vi "invert cluster.vi"(11 "subcarrier channels":T1) -> (2 "subcarrier channels out":T1)   [LabVIEW 2020]
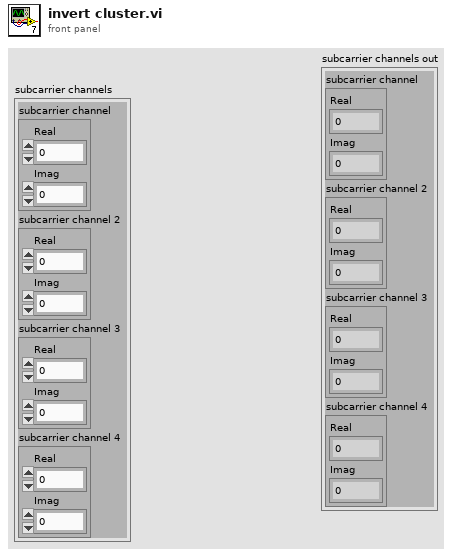
[diagram p1: front panel]
types:
  T1 = cluster{"subcarrier channel":cluster{"Real":fxp<+/-,25,4>, "Imag":fxp<+/-,25,4>}, "subcarrier channel 2":cluster{"Real":fxp<+/-,25,4>, "Imag":fxp<+/-,25,4>}, "subcarrier channel 3":cluster{"Real":fxp<+/-,25,4>, "Imag":fxp<+/-,25,4>}, "subcarrier channel 4":cluster{"Real":fxp<+/-,25,4>, "Imag":fxp<+/-,25,4>}}
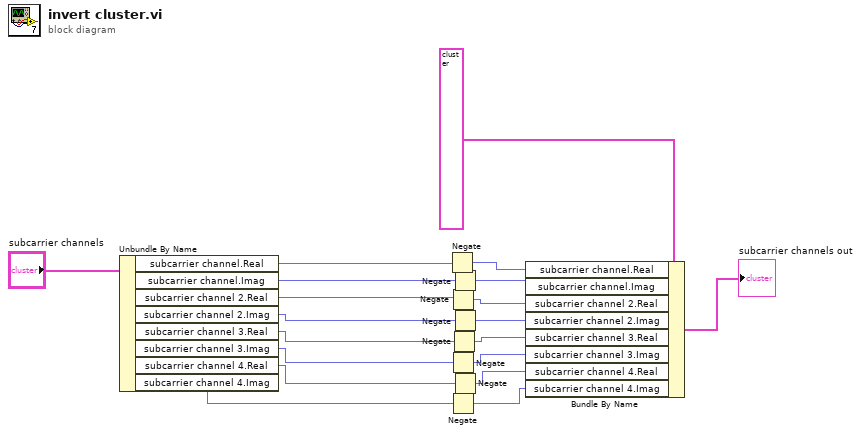
[diagram p0: block diagram]
diagram:
  n1 = Unbundle By Name("subcarrier channels") -> ("subcarrier channel.Real"=w14:fxp<+/-,25,4>, "subcarrier channel.Imag"=w15:fxp<+/-,25,4>, "subcarrier channel 2.Real"=w12:fxp<+/-,25,4>, "subcarrier channel 2.Imag"=w11:fxp<+/-,25,4>, "subcarrier channel 3.Real"=w10:fxp<+/-,25,4>, "subcarrier channel 3.Imag"=w9:fxp<+/-,25,4>, "subcarrier channel 4.Real"=w8:fxp<+/-,25,4>, "subcarrier channel 4.Imag"=w7:fxp<+/-,25,4>)
  n2 = Negate(x=w14) -> (-x=w16:fxp<+/-,25,4>)
  n3 = Negate(x=w12) -> (-x=w6:fxp<+/-,25,4>)
  n4 = Negate(x=w9) -> (-x=w3:fxp<+/-,25,4>)
  n5 = Negate(x=w7) -> (-x=w1:fxp<+/-,25,4>)
  n6 = Negate(x=w10) -> (-x=w4:fxp<+/-,25,4>)
  n7 = Negate(x=w15) -> (-x=w17:fxp<+/-,25,4>)
  n8 = Negate(x=w11) -> (-x=w5:fxp<+/-,25,4>)
  n9 = Negate(x=w8) -> (-x=w2:fxp<+/-,25,4>)
  n10 = Bundle By Name(cluster=T1 {"subcarrier channel"={"Real"=0.0, "Imag"=0.0}, "subcarrier channel 2"={"Real"=0.0, "Imag"=0.0}, "subcarrier channel 3"={"Real"=0.0, "Imag"=0.0}, "subcarrier channel 4"={"Real"=0.0, "Imag"=0.0}} ("subcarrier channels"), "subcarrier channel.Real"=w16, "subcarrier channel.Imag"=w17, "subcarrier channel 2.Real"=w6, "subcarrier channel 2.Imag"=w5, "subcarrier channel 3.Real"=w4, "subcarrier channel 3.Imag"=w3, "subcarrier channel 4.Real"=w2, "subcarrier channel 4.Imag"=w1) -> (→"subcarrier channels out":T1)
